vi "Read Database Files_CSV.vi"(8 "error in":errorcluster, 10 "Configuration":T1={"Name"="", "Description"="", "Diagnostics Basic Configuraiton"={"Database File"=path "", "CAN Interface"=enum."CAN0", "Baud Rate"=0, "Diagnostic Protocol"=enum."GMLAN", "Transport Protocol"=enum."ISO TP - Normal Mode", "Transmit ID"=0, "Receive ID"=0, "Transmit Extension"=0, "Receive Extension"=0, "Receive UUDT ID"=0, "Enable Stream"=TRUE, "VW TP Channel ID"=0, "Security"={"Type"=enum."None", "Source DLL Path"=path "", "Target DLL Path"=path "", "Security Level"=1, "Master Key"=""}}, "DIDs"={"Description"="", "Frames"=[]}, "Input PIDs"={"Description"="", "Frames"=[]}, "Output PIDs"={"Description"="", "Frames"=[]}, "DPIDs"={"Description"="", "DPIDs"=[]}, "DTC"={"Description"="", "DTC descriptor"={"DTC Byte Length"=2, "Status Byte Length"=1, "Add Data Byte Length"=1, "Byte Order"=enum."Motorola"}}, "NI 986x Support"={"Enable 986x"=FALSE, "RIO Device"=0, "Bitfile"=path ""}, "Commands"={"Description"=""}, "Status"={"Description"=""}, "IO Controls"={"Description"="", "IO Control Array"=[]}, "Routines"={"Description"="", "Routine Array"=[]}, "Output Memory"={"Description"="", "Frames"=[]}, "Input Memory"={"Description"="", "Frames"=[]}} {"Input Memory"."Frames"."Signals"."Byte Order" items=["Little Endian", "Big Endian"]; "Input Memory"."Frames"."Signals"."Data Type" items=["Signed", "Unsigned", "IEEE Float"]; "Output Memory"."Frames"."Signals"."Byte Order" items=["Little Endian", "Big Endian"]; "Output Memory"."Frames"."Signals"."Data Type" items=["Signed", "Unsigned", "IEEE Float"]; "Routines"."Routine Array"."Stop Parameters"."Response"."Byte Order" items=["Little Endian", "Big Endian"]; "Routines"."Routine Array"."Stop Parameters"."Response"."Data Type" items=["Signed", "Unsigned", "IEEE Float"]; "Routines"."Routine Array"."Stop Parameters"."Cmd"."Byte Order" items=["Little Endian", "Big Endian"]; "Routines"."Routine Array"."Stop Parameters"."Cmd"."Data Type" items=["Signed", "Unsigned", "IEEE Float"]; "Routines"."Routine Array"."Request Parameters"."Response"."Byte Order" items=["Little Endian", "Big Endian"]; "Routines"."Routine Array"."Request Parameters"."Response"."Data Type" items=["Signed", "Unsigned", "IEEE Float"]; "Routines"."Routine Array"."Request Parameters"."Cmd"."Byte Order" items=["Little Endian", "Big Endian"]; "Routines"."Routine Array"."Request Parameters"."Cmd"."Data Type" items=["Signed", "Unsigned", "IEEE Float"]; "Routines"."Routine Array"."Start Parameters"."Response"."Byte Order" items=["Little Endian", "Big Endian"]; "Routines"."Routine Array"."Start Parameters"."Response"."Data Type" items=["Signed", "Unsigned", "IEEE Float"]; "Routines"."Routine Array"."Start Parameters"."Cmd"."Byte Order" items=["Little Endian", "Big Endian"]; "Routines"."Routine Array"."Start Parameters"."Cmd"."Data Type" items=["Signed", "Unsigned", "IEEE Float"]; "IO Controls"."IO Control Array"."Signals"."Response"."Byte Order" items=["Little Endian", "Big Endian"]; "IO Controls"."IO Control Array"."Signals"."Response"."Data Type" items=["Signed", "Unsigned", "IEEE Float"]; "IO Controls"."IO Control Array"."Signals"."Cmd"."Byte Order" items=["Little Endian", "Big Endian"]; "IO Controls"."IO Control Array"."Signals"."Cmd"."Data Type" items=["Signed", "Unsigned", "IEEE Float"]; "Diagnostics Basic Configuraiton"."VW TP Channel ID" format="%.0x"; "Diagnostics Basic Configuraiton"."Receive UUDT ID" format="%.0x"; "Diagnostics Basic Configuraiton"."Receive Extension" format="%.0x"; "Diagnostics Basic Configuraiton"."Transmit Extension" format="%.0x"; "Diagnostics Basic Configuraiton"."Receive ID" format="%.0x"; "Diagnostics Basic Configuraiton"."Transmit ID" format="%.0x"; "DIDs"."Frames"."Signals"."Byte Order" items=["Little Endian", "Big Endian"]; "DIDs"."Frames"."Signals"."Data Type" items=["Signed", "Unsigned", "IEEE Float"]; "Input PIDs"."Frames"."Signals"."Byte Order" items=["Little Endian", "Big Endian"]; "Input PIDs"."Frames"."Signals"."Data Type" items=["Signed", "Unsigned", "IEEE Float"]; "Output PIDs"."Frames"."Signals"."Byte Order" items=["Little Endian", "Big Endian"]; "Output PIDs"."Frames"."Signals"."Data Type" items=["Signed", "Unsigned", "IEEE Float"]}, 11 "file (use dialog)":path) -> (0 "error out":errorcluster, 2 "Configuration 2":T1={"Name"="", "Description"="", "Diagnostics Basic Configuraiton"={"Database File"=path "", "CAN Interface"=enum."CAN0", "Baud Rate"=0, "Diagnostic Protocol"=enum."GMLAN", "Transport Protocol"=enum."ISO TP - Normal Mode", "Transmit ID"=0, "Receive ID"=0, "Transmit Extension"=0, "Receive Extension"=0, "Receive UUDT ID"=0, "Enable Stream"=TRUE, "VW TP Channel ID"=0, "Security"={"Type"=enum."None", "Source DLL Path"=path "", "Target DLL Path"=path "", "Security Level"=1, "Master Key"=""}}, "DIDs"={"Description"="", "Frames"=[]}, "Input PIDs"={"Description"="", "Frames"=[]}, "Output PIDs"={"Description"="", "Frames"=[]}, "DPIDs"={"Description"="", "DPIDs"=[]}, "DTC"={"Description"="", "DTC descriptor"={"DTC Byte Length"=2, "Status Byte Length"=1, "Add Data Byte Length"=1, "Byte Order"=enum."Motorola"}}, "NI 986x Support"={"Enable 986x"=FALSE, "RIO Device"=0, "Bitfile"=path ""}, "Commands"={"Description"=""}, "Status"={"Description"=""}, "IO Controls"={"Description"="", "IO Control Array"=[]}, "Routines"={"Description"="", "Routine Array"=[]}, "Output Memory"={"Description"="", "Frames"=[]}, "Input Memory"={"Description"="", "Frames"=[]}} {"Input Memory"."Frames"."Signals"."Byte Order" items=["Little Endian", "Big Endian"]; "Input Memory"."Frames"."Signals"."Data Type" items=["Signed", "Unsigned", "IEEE Float"]; "Output Memory"."Frames"."Signals"."Byte Order" items=["Little Endian", "Big Endian"]; "Output Memory"."Frames"."Signals"."Data Type" items=["Signed", "Unsigned", "IEEE Float"]; "Routines"."Routine Array"."Stop Parameters"."Response"."Byte Order" items=["Little Endian", "Big Endian"]; "Routines"."Routine Array"."Stop Parameters"."Response"."Data Type" items=["Signed", "Unsigned", "IEEE Float"]; "Routines"."Routine Array"."Stop Parameters"."Cmd"."Byte Order" items=["Little Endian", "Big Endian"]; "Routines"."Routine Array"."Stop Parameters"."Cmd"."Data Type" items=["Signed", "Unsigned", "IEEE Float"]; "Routines"."Routine Array"."Request Parameters"."Response"."Byte Order" items=["Little Endian", "Big Endian"]; "Routines"."Routine Array"."Request Parameters"."Response"."Data Type" items=["Signed", "Unsigned", "IEEE Float"]; "Routines"."Routine Array"."Request Parameters"."Cmd"."Byte Order" items=["Little Endian", "Big Endian"]; "Routines"."Routine Array"."Request Parameters"."Cmd"."Data Type" items=["Signed", "Unsigned", "IEEE Float"]; "Routines"."Routine Array"."Start Parameters"."Response"."Byte Order" items=["Little Endian", "Big Endian"]; "Routines"."Routine Array"."Start Parameters"."Response"."Data Type" items=["Signed", "Unsigned", "IEEE Float"]; "Routines"."Routine Array"."Start Parameters"."Cmd"."Byte Order" items=["Little Endian", "Big Endian"]; "Routines"."Routine Array"."Start Parameters"."Cmd"."Data Type" items=["Signed", "Unsigned", "IEEE Float"]; "IO Controls"."IO Control Array"."Signals"."Response"."Byte Order" items=["Little Endian", "Big Endian"]; "IO Controls"."IO Control Array"."Signals"."Response"."Data Type" items=["Signed", "Unsigned", "IEEE Float"]; "IO Controls"."IO Control Array"."Signals"."Cmd"."Byte Order" items=["Little Endian", "Big Endian"]; "IO Controls"."IO Control Array"."Signals"."Cmd"."Data Type" items=["Signed", "Unsigned", "IEEE Float"]; "Diagnostics Basic Configuraiton"."VW TP Channel ID" format="%.0x"; "Diagnostics Basic Configuraiton"."Receive UUDT ID" format="%.0x"; "Diagnostics Basic Configuraiton"."Receive Extension" format="%.0x"; "Diagnostics Basic Configuraiton"."Transmit Extension" format="%.0x"; "Diagnostics Basic Configuraiton"."Receive ID" format="%.0x"; "Diagnostics Basic Configuraiton"."Transmit ID" format="%.0x"; "DIDs"."Frames"."Signals"."Byte Order" items=["Little Endian", "Big Endian"]; "DIDs"."Frames"."Signals"."Data Type" items=["Signed", "Unsigned", "IEEE Float"]; "Input PIDs"."Frames"."Signals"."Byte Order" items=["Little Endian", "Big Endian"]; "Input PIDs"."Frames"."Signals"."Data Type" items=["Signed", "Unsigned", "IEEE Float"]; "Output PIDs"."Frames"."Signals"."Byte Order" items=["Little Endian", "Big Endian"]; "Output PIDs"."Frames"."Signals"."Data Type" items=["Signed", "Unsigned", "IEEE Float"]})   [LabVIEW 2019]
uses:
  Shared/Signal Parameters.ctl
  Shared/DTC Parameters.ctl
  Shared/DPID Periodic Rate.ctl
  Shared/DPID Parameters.ctl
  Shared/Frame Parameters.ctl
  Shared/Exported DPID Parameters.ctl
  Shared/Exported DPIDs Cluster.ctl
  Shared/Exported Frames Cluster.ctl
  Shared/Diagnostic Protocols.ctl
  Shared/CAN Interface.ctl
  Shared/Transport Protocols.ctl
  Shared/CAN Configuration.ctl
  <vilib>/Automotive Diagnostic Command Set/Diagnostic Protocols.llb/DTC Descriptor.ctl
  Shared/Exported DTC Cluster.ctl
  Shared/Exported 986x Support.ctl
  Shared/Exported Command Cluster.ctl
  Shared/Exported Status Cluster.ctl
  Shared/Exported Configuration.ctl
  Shared/Types/Security.ctl
  Shared/Diagnostics Addon Shared.lvlib
  Shared/IO Control Parameters.ctl
  Shared/Exported IO Control Cluster.ctl
  Shared/Input and Output Signal Parameters.ctl
  Shared/Routine Paramaters.ctl
  Shared/Exported Routines Cluster.ctl
  Shared/Types/Security.Type.ctl
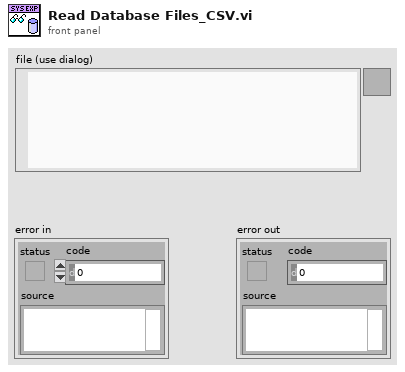
[diagram p1: front panel]
types:
  T1 = typedef "Diagnostics Addon System Explorer.lvlib/Exported Configuration.ctl" = cluster{"Name":string, "Description":string, "Diagnostics Basic Configuraiton":T2, "DIDs":T8, "Input PIDs":T8, "Output PIDs":T8, "DPIDs":T11, "DTC":T15, "NI 986x Support":T17, "Commands":T18, "Status":T19, "IO Controls":T20, "Routines":T23, "Output Memory":T8, "Input Memory":T8}
  T2 = typedef "Diagnostics Addon Shared.lvlib/CAN Configuration.ctl" = cluster{"Database File":path, "CAN Interface":T3, "Baud Rate":u32, "Diagnostic Protocol":T4, "Transport Protocol":T5, "Transmit ID":u32, "Receive ID":u32, "Transmit Extension":u8, "Receive Extension":u8, "Receive UUDT ID":u32, "Enable Stream":bool, "VW TP Channel ID":u32, "Security":T6}
  T3 = typedef "Diagnostics Addon Shared.lvlib/CAN Interface.ctl" = enum16{"CAN0", "CAN1", "CAN2", "CAN3", "CAN4", "CAN5", "CAN6", "CAN7", "CAN8", "CAN9", "CAN10", "CAN11", "CAN12", "CAN13", "CAN14", "CAN15", "CAN16", "CAN17", "CAN18", "CAN19", "CAN20", "CAN21", "CAN22", "CAN23", "CAN24", "CAN25", "CAN26", "CAN27", "CAN28", "CAN29", "CAN30", "CAN31", "CAN32", "CAN33", "CAN34", "CAN35", "CAN36", "CAN37", "CAN38", "CAN39", "CAN40", "CAN41", "CAN42", "CAN43", "CAN44", "CAN45", "CAN46", "CAN47", "CAN48", "CAN49", "CAN50", "CAN51", "CAN52", "CAN53", "CAN54", "CAN55", "CAN56", "CAN57", "CAN58", "CAN59", "CAN60", "CAN61", "CAN62", "CAN63", "CAN 256 (Virtual)", "CAN 257 (Virtual)"}
  T4 = typedef "Diagnostics Addon Shared.lvlib/Diagnostic Protocols.ctl" = enum16{"GMLAN", "KWP-2000", "UDS"}
  T5 = typedef "Diagnostics Addon Shared.lvlib/Transport Protocols.ctl" = enum16{"ISO TP - Normal Mode", "ISO TP - Mixed Mode", "VW TP 2.0", "Diagnostics on IP"}
  T6 = typedef "Diagnostics Addon Shared.lvlib/Security.ctl" = cluster{"Type":T7, "Source DLL Path":path, "Target DLL Path":path, "Security Level":u8, "Master Key":string}
  T7 = typedef "Diagnostics Addon Shared.lvlib/Security.Type.ctl" = enum16{"None", "DLL", "MasterKey"}
  T8 = typedef "Diagnostics Addon System Explorer.lvlib/Exported Frames Cluster.ctl" = cluster{"Description":string, "Frames":T9[]}
  T9 = typedef "Diagnostics Addon Shared.lvlib/Frame Parameters.ctl" = cluster{"Name":string, "Description":string, "ID":u16, "Signals":T10[]}
  T10 = typedef "Diagnostics Addon Shared.lvlib/Signal Parameters.ctl" = cluster{"Start Bit":u8, "Length":u8, "Scaling Factor":dbl, "Scaling Offset":dbl, "Minimum":dbl, "Maximum":dbl, "Data Type":u32, "Byte Order":u32, "Default Value":dbl, "Name":string, "Units":string, "Description":string}
  T11 = typedef "Diagnostics Addon System Explorer.lvlib/Exported DPIDs Cluster.ctl" = cluster{"Description":string, "DPIDs":T12[]}
  T12 = typedef "Diagnostics Addon System Explorer.lvlib/Exported DPID Parameters.ctl" = cluster{"Name":string, "Description":string, "DPID":T13}
  T13 = typedef "Diagnostics Addon Shared.lvlib/DPID Parameters.ctl" = cluster{"DPID ID":u8, "Speed":T14, "PIDs":u16[]}
  T14 = typedef "Diagnostics Addon Shared.lvlib/DPID Periodic Rate.ctl" = enum16{"Slow", "Medium", "Fast"}
  T15 = typedef "Diagnostics Addon System Explorer.lvlib/Exported DTC Cluster.ctl" = cluster{"Description":string, "DTC descriptor":T16}
  T16 = typedef "DTC Descriptor.ctl" = cluster{"DTC Byte Length":i32, "Status Byte Length":i32, "Add Data Byte Length":i32, "Byte Order":enum16{"Motorola", "Intel"}}
  T17 = typedef "Diagnostics Addon System Explorer.lvlib/Exported 986x Support.ctl" = cluster{"Enable 986x":bool, "RIO Device":u16, "Bitfile":path}
  T18 = typedef "Diagnostics Addon System Explorer.lvlib/Exported Command Cluster.ctl" = cluster{"Description":string}
  T19 = typedef "Diagnostics Addon System Explorer.lvlib/Exported Status Cluster.ctl" = cluster{"Description":string}
  T20 = typedef "Diagnostics Addon System Explorer.lvlib/Exported IO Control Cluster.ctl" = cluster{"Description":string, "IO Control Array":T21[]}
  T21 = typedef "Diagnostics Addon Shared.lvlib/IO Control Parameters.ctl" = cluster{"Name":string, "Description":string, "ID":u16, "Mode":u8, "Signals":T22}
  T22 = typedef "Diagnostics Addon Shared.lvlib/Input and Output Signal Parameters.ctl" = cluster{"Cmd":T10[], "Response":T10[]}
  T23 = typedef "Diagnostics Addon System Explorer.lvlib/Exported Routines Cluster.ctl" = cluster{"Description":string, "Routine Array":T24[]}
  T24 = typedef "Diagnostics Addon Shared.lvlib/Routine Paramaters.ctl" = cluster{"Name":string, "Description":string, "ID":u16, "Start Parameters":T22, "Request Parameters":T22, "Stop Parameters":T22}
  T25 = typedef "DTC Parameters.ctl" = cluster{"DTC Address":i32, "DTC Name":string, "DTC Description":string}
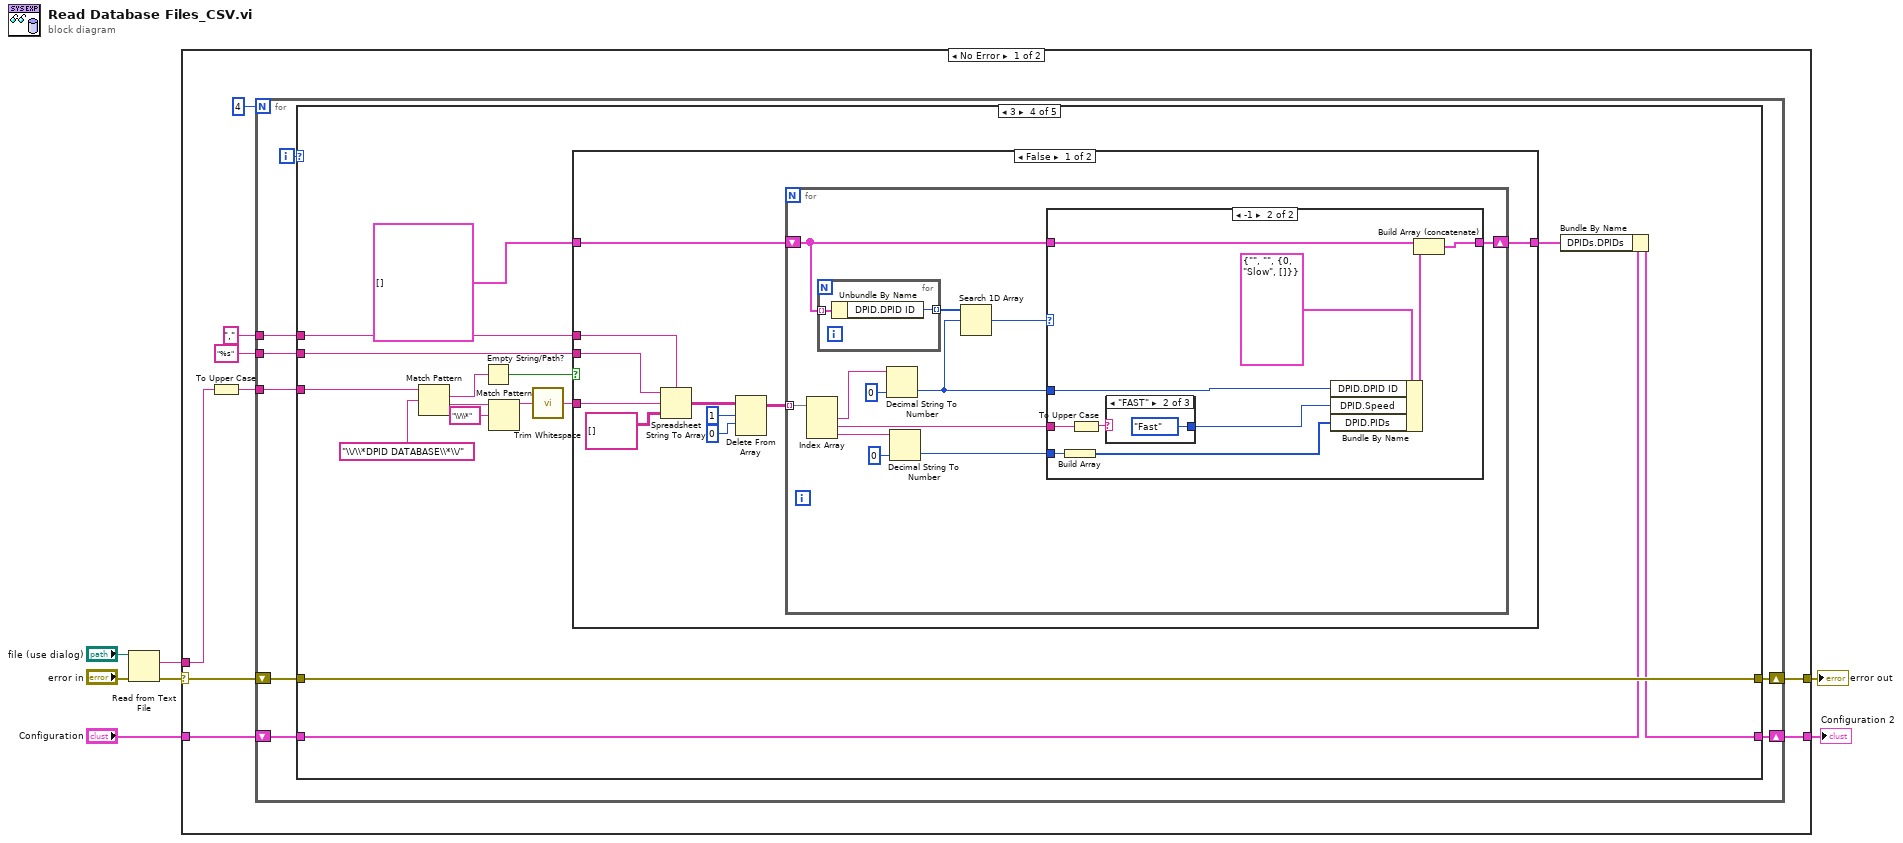
[diagram p0: block diagram]
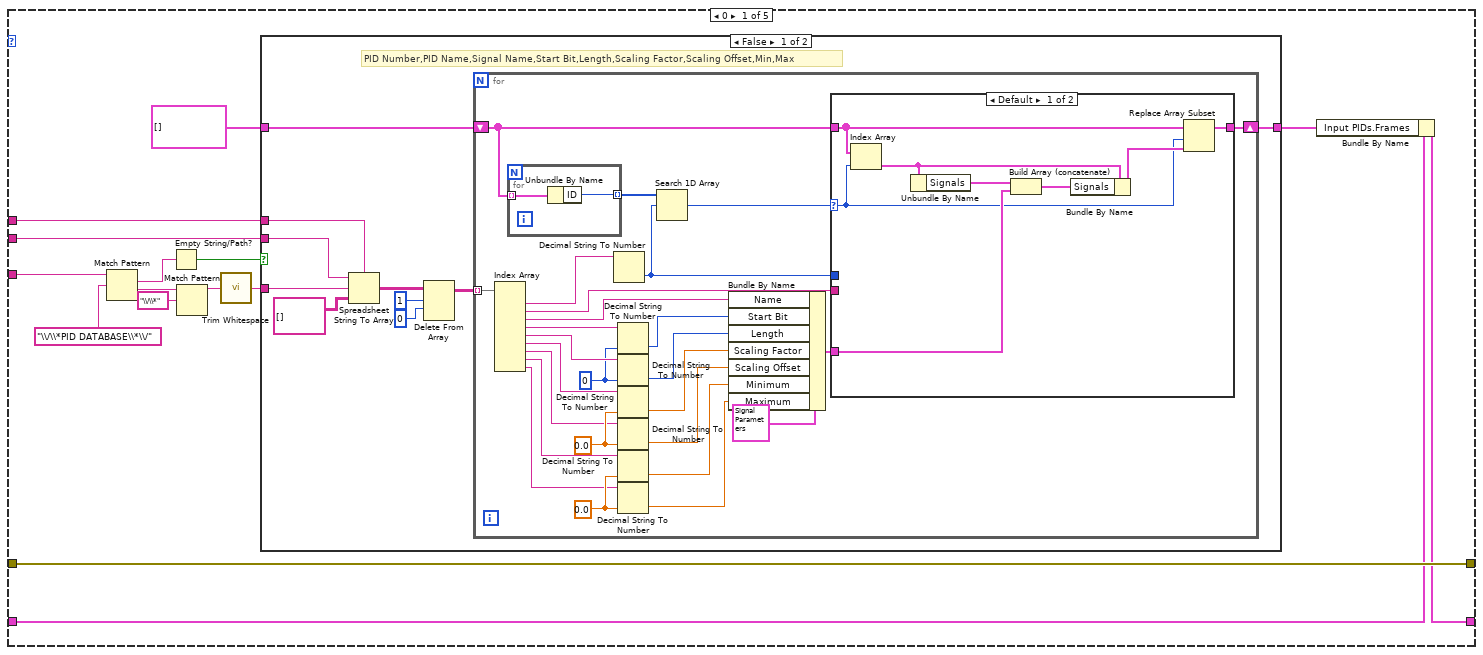
[diagram p2: hidden frame]
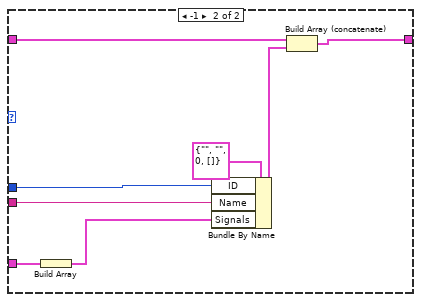
[diagram p3: hidden frame]
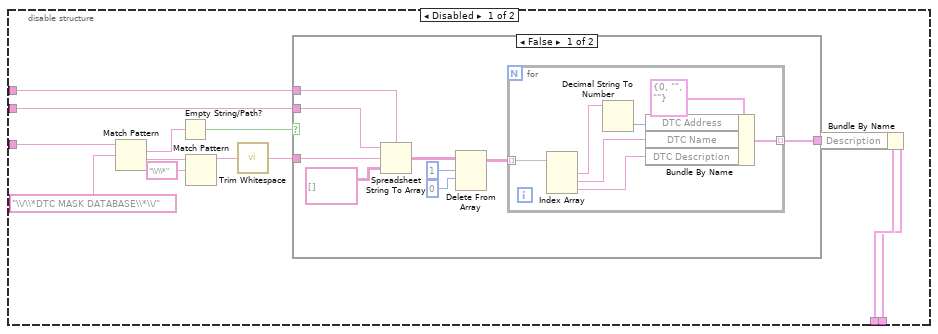
[diagram p6: hidden frame]
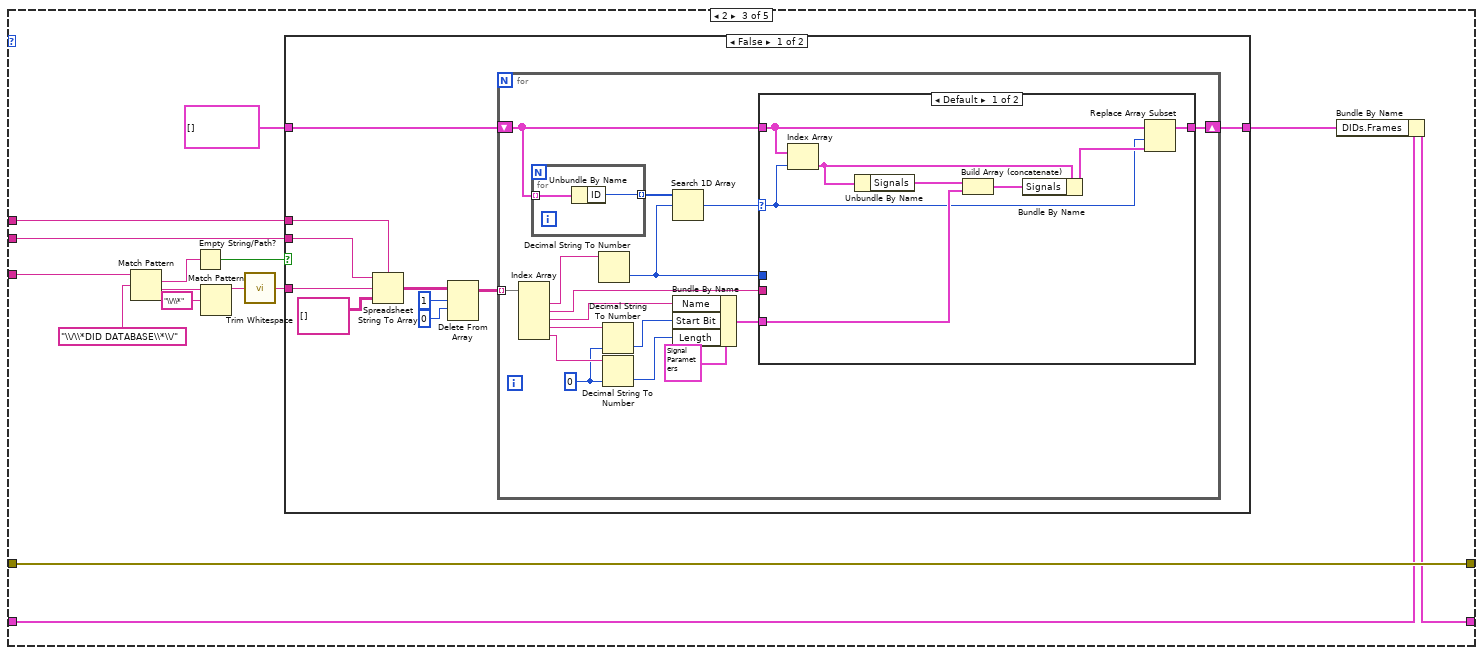
[diagram p8: hidden frame]
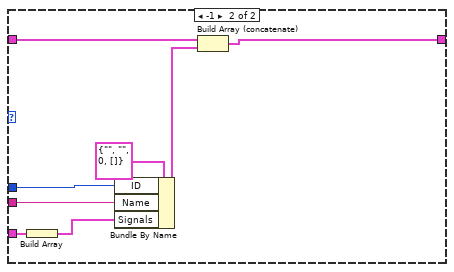
[diagram p9: hidden frame]
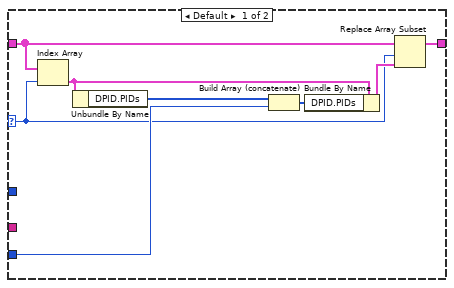
[diagram p11: hidden frame]
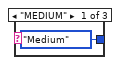
[diagram p12: hidden frame]
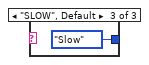
[diagram p13: hidden frame]
diagram:
  n1 = Read from Text File(file (use dialog)="file (use dialog)", error in="error in") -> (text=w5:string, error out=w4:errorcluster)  [unwired: 4 out]
  n2 = case shown="No Error" w4 {
    selector: w4 -> [w16 w255]
    tunnel: w5 -> [w15 _]
    tunnel: [w12 w255] -> w3
    tunnel: "Configuration" -> [w9 w254]
    tunnel: [w8 w254] -> w1
    frame No Error {
      n3 = To Upper Case(1:w15) -> (0:w14:string)
      n4 = for {
        N: 4 -> [_]
        shift-right: [w22] -> w12
        shift-left: w16 -> [w24]
        tunnel: w14 -> [w23]
        tunnel: "," ("delimiter (Tab)") -> [w20]
        tunnel: "%s" ("format string") -> [w19]
        shift-right: [w17] -> w8
        shift-left: w9 -> [w18]
        i -> [w21]
        n5 = case shown="3" w21 {
          tunnel: w24 -> [w35 w99 w141 w201 w253]
          tunnel: w23 -> [w39 w100 w145 w205 _]
          tunnel: [w35 w99 w141 w201 w253] -> w22
          tunnel: w20 -> [w29 w98 w135 w195 _]
          tunnel: w19 -> [w30 w97 w136 w196 _]
          tunnel: w18 -> [w27 w96 w134 w193 w252]
          tunnel: [w25 w95 w133 w191 w252] -> w17
          frame 0 {
            n6 = Match Pattern(string=w39, regular expression="\\/\\*PID DATABASE\\*\\/") -> (match substring=w34:string, after substring=w37:string)  [unwired: 1 in, 2 out]
            n7 = Empty String/Path?(string/path=w34) -> (empty?=w31:bool)
            n8 = Match Pattern(string=w37, regular expression="\\/\\*") -> (before substring=w33:string)  [unwired: 1 in, 3 out]
            n9 = call <vilib>:"Trim Whitespace.vi"("string"=w33) -> ("trimmed string"=w32:string)  [unwired: 1 in]
            n10 = case shown="False" w31 {
              tunnel: w32 -> [w48 _]
              tunnel: w29 -> [w47 _]
              tunnel: w30 -> [w46 _]
              tunnel: [w42 w94] -> w26
              tunnel: T9[] [] ("Array") -> [w41 w94]
              frame False {
                # "PID Number,PID Name,Signal Name,Start Bit,Length,Scaling Factor,Scaling Offset,Min,Max"
                n11 = Spreadsheet String To Array(delimiter (Tab)=w47, format string=w46, spreadsheet string=w48, array type (2D Dbl)=string[][] []) -> (array=w45:string[][])
                n12 = Delete From Array(array=w45, length=1, index (row)=0 ("index")) -> (array with subset deleted=w40:string[][])  [unwired: 1 in, 1 out]
                n13 = for {
                  tunnel: w40 -> [w75] mode=indexing
                  shift-right: [w61] -> w42
                  shift-left: w41 -> [w62]
                  w55 = 0.0 ("default (0 I32)")
                  w60 = 0.0 ("default (0 I32)")
                  w70 = u8 0 ("default (0 I32)")
                  n14 = Index Array(array=w75) -> (element #1=w74:string, element #2=w73:string, element #3=w66:string, element #4=w72:string, element #5=w71:string, element #6=w59:string, element #7=w58:string, element #8=w54:string, element #9=w53:string)  [unwired: 9 in]
                  n15 = for {
                    tunnel: w62 -> [w93] mode=indexing
                    tunnel: [w92] -> w69 mode=indexing
                    n16 = Unbundle By Name(w93) -> ("ID"=w92:u16)
                  }
                  n17 = Decimal String To Number(string=w74) -> (number=w64:i32)  [unwired: 2 in, 1 out]
                  n18 = Decimal String To Number(string=w72, default (0L)=w70) -> (number=w67:u8)  [unwired: 1 in, 1 out]
                  n19 = Decimal String To Number(string=w71, default (0L)=w70) -> (number=w68:u8)  [unwired: 1 in, 1 out]
                  n20 = Decimal String To Number(string=w59, default (0L)=w60) -> (number=w57:dbl)  [unwired: 1 in, 1 out]
                  n21 = Decimal String To Number(string=w58, default (0L)=w60) -> (number=w56:dbl)  [unwired: 1 in, 1 out]
                  n22 = Decimal String To Number(string=w54, default (0L)=w55) -> (number=w52:dbl)  [unwired: 1 in, 1 out]
                  n23 = Decimal String To Number(string=w53, default (0L)=w55) -> (number=w51:dbl)  [unwired: 1 in, 1 out]
                  n24 = Search 1D Array(1D array=w69, element=w64) -> (index of element=w63:i32)  [unwired: 1 in]
                  n25 = Bundle By Name(cluster=T10 {"Start Bit"=0, "Length"=0, "Scaling Factor"=0.0, "Scaling Offset"=0.0, "Minimum"=0.0, "Maximum"=0.0, "Data Type"=0, "Byte Order"=0, "Default Value"=0.0, "Name"="", "Units"="", "Description"=""} ("Signal Parameters"), "Name"=w66, "Start Bit"=w67, "Length"=w68, "Scaling Factor"=w57, "Scaling Offset"=w56, "Minimum"=w52, "Maximum"=w51) -> (w65:T10)
                  n26 = case shown="Default" w63 {
                    selector: w63 -> [w76 _]
                    tunnel: w73 -> [_ w91]
                    tunnel: w65 -> [w80 w90]
                    tunnel: w64 -> [_ w88]
                    tunnel: w62 -> [w82 w87]
                    tunnel: [w83 w85] -> w61
                    frame Default {
                      n27 = Index Array(array=w82, index=w76) -> (element=w79:T9)
                      n28 = Unbundle By Name(w79) -> ("Signals"=w81:T10[])
                      n29 = Build Array (concatenate)(w81, w80) -> (w78:T10[])
                      n30 = Bundle By Name(cluster=w79, "Signals"=w78) -> (w77:T9)
                      n31 = Replace Array Subset(array=w82, new element=w77, index=w76) -> (w83:T9[])
                    }
                    frame -1 {
                      n32 = Build Array(w90) -> (w89:T10[])
                      n33 = Bundle By Name(cluster=T9 {"Name"="", "Description"="", "ID"=0, "Signals"=[]} ("DIDPID"), "ID"=w88, "Name"=w91, "Signals"=w89) -> (w86:T9)
                      n34 = Build Array (concatenate)(w87, w86) -> (w85:T9[])
                    }
                  }
                }
              }
              frame True {
              }
            }
            n35 = Bundle By Name(cluster=w27, "Input PIDs.Frames"=w26) -> (w25:T1)
          }
          frame 1 {
            n36 = disable-structure shown="Enabled" {
              disable-tunnel: w100 -> [w113 _]
              disable-tunnel: w98 -> [w105 _]
              disable-tunnel: w97 -> [w104 _]
              disable-tunnel: w96 -> [w103 w130]
              disable-tunnel: [w101 w130] -> w95
              frame Disabled {
                n37 = Match Pattern(string=w113, regular expression="\\/\\*DTC MASK DATABASE\\*\\/") -> (match substring=w108:string, after substring=w111:string)  [unwired: 1 in, 2 out]
                n38 = Empty String/Path?(string/path=w108) -> (empty?=w106:bool)
                n39 = Match Pattern(string=w111, regular expression="\\/\\*") -> (before substring=w109:string)  [unwired: 1 in, 3 out]
                n40 = call <vilib>:"Trim Whitespace.vi"("string"=w109) -> ("trimmed string"=w107:string)  [unwired: 1 in]
                n41 = case shown="False" w106 {
                  tunnel: w107 -> [w121 _]
                  tunnel: w105 -> [w120 _]
                  tunnel: w104 -> [w119 _]
                  tunnel: [w115 _] -> w102
                  frame False {
                    n42 = Spreadsheet String To Array(delimiter (Tab)=w120, format string=w119, spreadsheet string=w121, array type (2D Dbl)=string[][] []) -> (array=w118:string[][])
                    n43 = Delete From Array(array=w118, length=1, index (row)=0 ("index")) -> (array with subset deleted=w114:string[][])  [unwired: 1 in, 1 out]
                    n44 = for {
                      tunnel: w114 -> [w128] mode=indexing
                      tunnel: [w124] -> w115 mode=indexing
                      n45 = Index Array(array=w128) -> (element #1=w129:string, element #2=w125:string, element #3=w126:string)  [unwired: 3 in]
                      n46 = Decimal String To Number(string=w129) -> (number=w127:i32)  [unwired: 2 in, 1 out]
                      n47 = Bundle By Name(cluster=T25 {"DTC Address"=0, "DTC Name"="", "DTC Description"=""}, "DTC Address"=w127, "DTC Name"=w125, "DTC Description"=w126) -> (w124:T25)
                    }
                  }
                  frame True {
                  }
                }
                n48 = Bundle By Name(cluster=w103, "Description"=w102) -> (w101:T1)
              }
              frame Enabled {
              }
            }
          }
          frame 2 {
            n49 = Match Pattern(string=w145, regular expression="\\/\\*DID DATABASE\\*\\/") -> (match substring=w140:string, after substring=w143:string)  [unwired: 1 in, 2 out]
            n50 = Empty String/Path?(string/path=w140) -> (empty?=w137:bool)
            n51 = Match Pattern(string=w143, regular expression="\\/\\*") -> (before substring=w139:string)  [unwired: 1 in, 3 out]
            n52 = call <vilib>:"Trim Whitespace.vi"("string"=w139) -> ("trimmed string"=w138:string)  [unwired: 1 in]
            n53 = case shown="False" w137 {
              tunnel: w138 -> [w154 _]
              tunnel: w135 -> [w153 _]
              tunnel: w136 -> [w152 _]
              tunnel: [w148 w190] -> w131
              tunnel: T9[] [] ("DIDs.DIDPID Array") -> [w147 w190]
              frame False {
                n54 = Spreadsheet String To Array(delimiter (Tab)=w153, format string=w152, spreadsheet string=w154, array type (2D Dbl)=string[][] []) -> (array=w151:string[][])
                n55 = Delete From Array(array=w151, length=1, index (row)=0 ("index")) -> (array with subset deleted=w146:string[][])  [unwired: 1 in, 1 out]
                n56 = for {
                  tunnel: w146 -> [w171] mode=indexing
                  shift-right: [w157] -> w148
                  shift-left: w147 -> [w158]
                  w166 = u8 0 ("default (0 I32)")
                  n57 = Index Array(array=w171) -> (element #1=w170:string, element #2=w169:string, element #3=w162:string, element #4=w168:string, element #5=w167:string)  [unwired: 5 in]
                  n58 = for {
                    tunnel: w158 -> [w189] mode=indexing
                    tunnel: [w188] -> w165 mode=indexing
                    n59 = Unbundle By Name(w189) -> ("ID"=w188:u16)
                  }
                  n60 = Decimal String To Number(string=w170) -> (number=w160:i32)  [unwired: 2 in, 1 out]
                  n61 = Decimal String To Number(string=w168, default (0L)=w166) -> (number=w163:u8)  [unwired: 1 in, 1 out]
                  n62 = Decimal String To Number(string=w167, default (0L)=w166) -> (number=w164:u8)  [unwired: 1 in, 1 out]
                  n63 = Search 1D Array(1D array=w165, element=w160) -> (index of element=w159:i32)  [unwired: 1 in]
                  n64 = Bundle By Name(cluster=T10 {"Start Bit"=0, "Length"=0, "Scaling Factor"=0.0, "Scaling Offset"=0.0, "Minimum"=0.0, "Maximum"=0.0, "Data Type"=0, "Byte Order"=0, "Default Value"=0.0, "Name"="", "Units"="", "Description"=""}, "Name"=w162, "Start Bit"=w163, "Length"=w164) -> (w161:T10)
                  n65 = case shown="Default" w159 {
                    selector: w159 -> [w172 _]
                    tunnel: w169 -> [_ w187]
                    tunnel: w161 -> [w176 w186]
                    tunnel: w160 -> [_ w184]
                    tunnel: w158 -> [w178 w183]
                    tunnel: [w179 w181] -> w157
                    frame Default {
                      n66 = Index Array(array=w178, index=w172) -> (element=w175:T9)
                      n67 = Unbundle By Name(w175) -> ("Signals"=w177:T10[])
                      n68 = Build Array (concatenate)(w177, w176) -> (w174:T10[])
                      n69 = Bundle By Name(cluster=w175, "Signals"=w174) -> (w173:T9)
                      n70 = Replace Array Subset(array=w178, new element=w173, index=w172) -> (w179:T9[])
                    }
                    frame -1 {
                      n71 = Build Array(w186) -> (w185:T10[])
                      n72 = Bundle By Name(cluster=T9 {"Name"="", "Description"="", "ID"=0, "Signals"=[]} ("DIDPID"), "ID"=w184, "Name"=w187, "Signals"=w185) -> (w182:T9)
                      n73 = Build Array (concatenate)(w183, w182) -> (w181:T9[])
                    }
                  }
                }
              }
              frame True {
              }
            }
            n74 = Bundle By Name(cluster=w134, "DIDs.Frames"=w131) -> (w133:T1)
          }
          frame 3 {
            n75 = Match Pattern(string=w205, regular expression="\\/\\*DPID DATABASE\\*\\/") -> (match substring=w200:string, after substring=w203:string)  [unwired: 1 in, 2 out]
            n76 = Empty String/Path?(string/path=w200) -> (empty?=w197:bool)
            n77 = Match Pattern(string=w203, regular expression="\\/\\*") -> (before substring=w199:string)  [unwired: 1 in, 3 out]
            n78 = call <vilib>:"Trim Whitespace.vi"("string"=w199) -> ("trimmed string"=w198:string)  [unwired: 1 in]
            n79 = case shown="False" w197 {
              tunnel: w198 -> [w214 _]
              tunnel: w195 -> [w213 _]
              tunnel: w196 -> [w212 _]
              tunnel: [w208 w251] -> w192
              tunnel: T12[] [] ("DPIDs") -> [w207 w251]
              frame False {
                n80 = Spreadsheet String To Array(delimiter (Tab)=w213, format string=w212, spreadsheet string=w214, array type (2D Dbl)=string[][] []) -> (array=w211:string[][])
                n81 = Delete From Array(array=w211, length=1, index (row)=0 ("index")) -> (array with subset deleted=w206:string[][])  [unwired: 1 in, 1 out]
                n82 = for {
                  tunnel: w206 -> [w227] mode=indexing
                  shift-right: [w220] -> w208
                  shift-left: w207 -> [w221]
                  n83 = Index Array(array=w227) -> (element #1=w226:string, element #2=w225:string, element #3=w219:string)  [unwired: 3 in]
                  n84 = for {
                    tunnel: w221 -> [w250] mode=indexing
                    tunnel: [w249] -> w224 mode=indexing
                    n85 = Unbundle By Name(w250) -> ("DPID.DPID ID"=w249:u8)
                  }
                  n86 = Decimal String To Number(string=w226, default (0L)=u8 0 ("default (0 I32)")) -> (number=w223:u8)  [unwired: 1 in, 1 out]
                  n87 = Decimal String To Number(string=w219, default (0L)=u16 0 ("default (0 I32)")) -> (number=w218:u16)  [unwired: 1 in, 1 out]
                  n88 = Search 1D Array(1D array=w224, element=w223) -> (index of element=w222:i32)  [unwired: 1 in]
                  n89 = case shown="-1" w222 {
                    selector: w222 -> [w228 _]
                    tunnel: w225 -> [_ w238]
                    tunnel: w218 -> [w232 w245]
                    tunnel: w223 -> [_ w243]
                    tunnel: w221 -> [w234 w242]
                    tunnel: [w235 w240] -> w220
                    frame Default {
                      n90 = Index Array(array=w234, index=w228) -> (element=w231:T12)
                      n91 = Unbundle By Name(w231) -> ("DPID.PIDs"=w233:u16[])
                      n92 = Build Array (concatenate)(w233, w232) -> (w230:u16[])
                      n93 = Bundle By Name(cluster=w231, "DPID.PIDs"=w230) -> (w229:T12)
                      n94 = Replace Array Subset(array=w234, new element=w229, index=w228) -> (w235:T12[])
                    }
                    frame -1 {
                      n95 = Build Array(w245) -> (w244:u16[])
                      n96 = To Upper Case(1:w238) -> (0:w239:string)
                      n97 = case shown="\"FAST\"" w239 {
                        tunnel: [DPID_Periodic_Rate."Medium" ("Speed") DPID_Periodic_Rate."Fast" ("Speed") DPID_Periodic_Rate."Slow" ("Speed")] -> w237
                        frame "MEDIUM" {
                        }
                        frame "FAST" {
                        }
                        frame "SLOW", Default {
                        }
                      }
                      n98 = Bundle By Name(cluster=T12 {"Name"="", "Description"="", "DPID"={"DPID ID"=0, "Speed"=enum."Slow", "PIDs"=[]}} ("DPID"), "DPID.DPID ID"=w243, "DPID.Speed"=w237, "DPID.PIDs"=w244) -> (w241:T12)
                      n99 = Build Array (concatenate)(w242, w241) -> (w240:T12[])
                    }
                  }
                }
              }
              frame True {
              }
            }
            n100 = Bundle By Name(cluster=w193, "DPIDs.DPIDs"=w192) -> (w191:T1)
          }
          frame Default {
          }
        }
      }
    }
    frame Error {
    }
  }
  "error out" <- w3
  "Configuration 2" <- w1
